vi "button_test.vi"() -> ()   [LabVIEW 2010]
panel:
  in  "Boolesch":bool
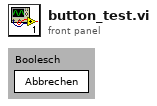
[diagram p1: front panel]
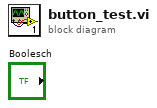
[diagram p0: block diagram]
diagram:
